vi "Dresden Edit Recipe(in).vi"() -> ()   [LabVIEW 2009] (continued)
          n32 = Scan Value(string=w38, format string="") -> (value=w237:dbl)  [unwired: 1 in, 1 out]
          n33 = Scan Value(string=w40, format string="") -> (value=w249:dbl)  [unwired: 1 in, 1 out]
          n34 = Scan Value(string=w43, format string="") -> (value=w365:dbl)  [unwired: 1 in, 1 out]
          n35 = Scan Value(string=w44, format string="") -> (value=w366:dbl)  [unwired: 1 in, 1 out]
          n36 = Equal?(x="Active", y=w53) -> (x = y?=w134:bool)
          n37 = Scan Value(string=w42, format string="") -> (value=w364:dbl)  [unwired: 1 in, 1 out]
          n38 = Scan Value(string=w35, format string="") -> (value=w231:dbl)  [unwired: 1 in, 1 out]
          n39 = Scan Value(string=w36, format string="") -> (value=w234:dbl)  [unwired: 1 in, 1 out]
          n40 = Scan Value(string=w34, format string="") -> (value=w230:dbl)  [unwired: 1 in, 1 out]
          n41 = Scan Value(string=w56, format string="") -> (value=w387:dbl)  [unwired: 1 in, 1 out]
          n42 = Scan Value(string=w52, format string="") -> (value=w380:dbl)  [unwired: 1 in, 1 out]
          n43 = Scan Value(string=w55, format string="") -> (value=w386:dbl)  [unwired: 1 in, 1 out]
          n44 = case shown="False" w131 {
            frame #0 {
              n45 = local write "Thickness_Monitor_Active"(FALSE ("Thickness_Monitor_Active")) -> ()
            }
            frame #1 {
              n46 = local write "Thickness_Monitor_Active"(TRUE ("Thickness_Monitor_Active")) -> ()
            }
          }
          n47 = Scan Value(string=w51, format string="") -> (value=w379:dbl)  [unwired: 1 in, 1 out]
          n48 = Scan Value(string=w47, format string="") -> (value=w372:dbl)  [unwired: 1 in, 1 out]
          n49 = Scan Value(string=w48, format string="") -> (value=w373:dbl)  [unwired: 1 in, 1 out]
          n50 = case shown="1" w241 {
            frame #0 {
            }
            frame #1 {
              n51 = local write "R_First_stop_selection"(enum32{"Chamber II", "Chamber III"}."Chamber II" ("R_First_stop_selection")) -> ()
            }
            frame #2 {
              n52 = local write "R_First_stop_selection"(enum32{"Chamber II", "Chamber III"}."Chamber III" ("R_First_stop_selection")) -> ()
            }
          }
          n53 = Scan Value(string=w54, format string="") -> (value=w385:dbl)  [unwired: 1 in, 1 out]
          n54 = Scan Value(string=w46, format string="") -> (value=w371:dbl)  [unwired: 1 in, 1 out]
          n55 = case shown="False" w429 {
            frame #0 {
              n56 = local write "R Cmb Step2 Coating Power Active"(FALSE ("R Cmb Step2 Coating Power Active")) -> ()
            }
            frame #1 {
              n57 = local write "R Cmb Step2 Coating Power Active"(TRUE ("R Cmb Step2 Coating Power Active")) -> ()
            }
          }
          n58 = Scan Value(string=w50, format string="") -> (value=w378:dbl)  [unwired: 1 in, 1 out]
          n59 = case shown="False" w421 {
            frame #0 {
              n60 = local write "R Cmb Step3 Coating Power Active"(FALSE ("R Cmb Step3 Coating Power Active")) -> ()
            }
            frame #1 {
              n61 = local write "R Cmb Step3 Coating Power Active"(TRUE ("R Cmb Step3 Coating Power Active")) -> ()
            }
          }
          n62 = Scan Value(string=w60, format string="") -> (value=w394:dbl)  [unwired: 1 in, 1 out]
          n63 = Scan Value(string=w59, format string="") -> (value=w393:dbl)  [unwired: 1 in, 1 out]
          n64 = Equal?(x="Active", y=w45) -> (x = y?=w133:bool)
          n65 = Scan Value(string=w58, format string="") -> (value=w392:dbl)  [unwired: 1 in, 1 out]
          n66 = Equal?(x="Active", y=w49) -> (x = y?=w132:bool)
          n67 = case shown="False" w413 {
            frame #0 {
              n68 = local write "R Cmb Step4 Coating Power Active"(FALSE ("R Cmb Step4 Coating Power Active")) -> ()
            }
            frame #1 {
              n69 = local write "R Cmb Step4 Coating Power Active"(TRUE ("R Cmb Step4 Coating Power Active")) -> ()
            }
          }
          n70 = case shown="False" w405 {
            frame #0 {
              n71 = local write "R Cmb Step5 Coating Power Active"(FALSE ("R Cmb Step5 Coating Power Active")) -> ()
            }
            frame #1 {
              n72 = local write "R Cmb Step5 Coating Power Active"(TRUE ("R Cmb Step5 Coating Power Active")) -> ()
            }
          }
          n73 = case shown="False" w136 {
            frame #0 {
              n74 = local write "R Cmb Step6 Coating Power Active"(FALSE ("R Cmb Step6 Coating Power Active")) -> ()
            }
            frame #1 {
              n75 = local write "R Cmb Step6 Coating Power Active"(TRUE ("R Cmb Step6 Coating Power Active")) -> ()
            }
          }
          n76 = Scan Value(string=w68, format string="") -> (value=w409:dbl)  [unwired: 1 in, 1 out]
          n77 = Scan Value(string=w67, format string="") -> (value=w408:dbl)  [unwired: 1 in, 1 out]
          n78 = Scan Value(string=w64, format string="") -> (value=w401:dbl)  [unwired: 1 in, 1 out]
          n79 = Scan Value(string=w81, format string="") -> (value=w433:dbl)  [unwired: 1 in, 1 out]
          n80 = Scan Value(string=w78, format string="") -> (value=w431:dbl)  [unwired: 1 in, 1 out]
          n81 = Scan Value(string=w63, format string="") -> (value=w400:dbl)  [unwired: 1 in, 1 out]
          n82 = case shown="True" w135 {
            frame #0 {
              n83 = local write "R Cmb Step7 Coating Power Active"(FALSE ("R Cmb Step7 Coating Power Active")) -> ()
            }
            frame #1 {
              n84 = local write "R Cmb Step7 Coating Power Active"(TRUE ("R Cmb Step7 Coating Power Active")) -> ()
            }
          }
          n85 = Scan Value(string=w66, format string="") -> (value=w407:dbl)  [unwired: 1 in, 1 out]
          n86 = Scan Value(string=w80, format string="") -> (value=w432:dbl)  [unwired: 1 in, 1 out]
          n87 = Scan Value(string=w62, format string="") -> (value=w399:dbl)  [unwired: 1 in, 1 out]
          n88 = Scan Value(string=w72, format string="") -> (value=w419:dbl)  [unwired: 1 in, 1 out]
          n89 = Scan Value(string=w71, format string="") -> (value=w416:dbl)  [unwired: 1 in, 1 out]
          n90 = case shown="True" w134 {
            frame #0 {
              n91 = local write "R Cmb Step8 Coating Power Active"(FALSE ("R Cmb Step8 Coating Power Active")) -> ()
            }
            frame #1 {
              n92 = local write "R Cmb Step8 Coating Power Active"(TRUE ("R Cmb Step8 Coating Power Active")) -> ()
            }
          }
          n93 = local write "R Cmb Number of cycle"(w249) -> ()
          n94 = Scan Value(string=w76, format string="") -> (value=w425:dbl)  [unwired: 1 in, 1 out]
          n95 = Scan Value(string=w74, format string="") -> (value=w423:dbl)  [unwired: 1 in, 1 out]
          n96 = Scan Value(string=w70, format string="") -> (value=w415:dbl)  [unwired: 1 in, 1 out]
          n97 = Scan Value(string=w75, format string="") -> (value=w424:dbl)  [unwired: 1 in, 1 out]
          n98 = case shown="True" w133 {
            frame #0 {
              n99 = local write "R Cmb Step10 Coating Power Active"(FALSE ("R Cmb Step10 Coating Power Active")) -> ()
            }
            frame #1 {
              n100 = local write "R Cmb Step10 Coating Power Active"(TRUE ("R Cmb Step10 Coating Power Active")) -> ()
            }
          }
          n101 = local write "R Cmb Ch2 Step10 Coating Power"(w366) -> ()
          n102 = case shown="True" w132 {
            frame #0 {
              n103 = local write "R Cmb Step9 Coating Power Active"(FALSE ("R Cmb Step9 Coating Power Active")) -> ()
            }
            frame #1 {
              n104 = local write "R Cmb Step9 Coating Power Active"(TRUE ("R Cmb Step9 Coating Power Active")) -> ()
            }
          }
          n105 = local write "R Cmb Ch3 Step10 Coating Power"(w365) -> ()
          n106 = local write "R Toooling_factor"(w230) -> ()
          n107 = local write "R Cmb Ch2 Step9 Coating Power"(w373) -> ()
          n108 = local write "R Cmb Ch3 Step9 Coating Power"(w372) -> ()
          n109 = local write "R Cmb Ch3 Step6 Coating Power"(w393) -> ()
          n110 = local write "R Cmb Ch3 Step8 Coating Power"(w379) -> ()
          n111 = local write "R Set Pressure mtorr"(w237) -> ()
          n112 = local write "R Cmb Ch3 Step1 Coating Power"(w432) -> ()
          n113 = local write "R Z_factor"(w231) -> ()
          n114 = local write "R Argon Flow sccm"(w238) -> ()
          n115 = local write "R Cmb Interval length 10"(w364) -> ()
          n116 = local write "R Cmb Ch2 Step7 Coating Power"(w387) -> ()
          n117 = local write "R Cmb Ch3 Step7 Coating Power"(w386) -> ()
          n118 = local write "R Cmb Ch2 Step1 Coating Power"(w433) -> ()
          n119 = local write "R Cmb Interval length 1"(w431) -> ()
          n120 = local write "R Material_density"(w234) -> ()
          n121 = local write "R Cmb Ch2 Step6 Coating Power"(w394) -> ()
          n122 = local write "R Cmb Ch2 Step8 Coating Power"(w380) -> ()
          n123 = local write "R Cmb Ch2 Step5 Coating Power"(w401) -> ()
          n124 = local write "R Cmb Ch3 Step5 Coating Power"(w400) -> ()
          n125 = local write "R Cmb Interval length 9"(w371) -> ()
          n126 = local write "R Cmb Ch2 Step2 Coating Power"(w425) -> ()
          n127 = local write "R Cmb Interval length 8"(w378) -> ()
          n128 = local write "R Cmb Ch3 Step2 Coating Power"(w424) -> ()
          n129 = local write "R Cmb Ch2 Step4 Coating Power"(w409) -> ()
          n130 = local write "R Cmb Ch3 Step3 Coating Power"(w416) -> ()
          n131 = local write "R Cmb Interval length 3"(w415) -> ()
          n132 = local write "R Cmb Interval length 6"(w392) -> ()
          n133 = local write "R Cmb Ch3 Step4 Coating Power"(w408) -> ()
          n134 = local write "R Cmb Interval length 5"(w399) -> ()
          n135 = local write "R Cmb Interval length 7"(w385) -> ()
          n136 = local write "R Cmb Ch2 Step3 Coating Power"(w419) -> ()
          n137 = local write "R Cmb Interval length 2"(w423) -> ()
          n138 = Scan Value(string=w82, format string="") -> (value=w434:dbl)  [unwired: 1 in, 1 out]
          n139 = local write "R Cmb Interval length 4"(w407) -> ()
          n140 = Scan Value(string=w84, format string="") -> (value=w435:dbl)  [unwired: 1 in, 1 out]
          n141 = local write "R Cmb Ch3 Target material"(w83) -> ()
          n142 = local write "R_Cmb_Ch3_Web_speed"(w434) -> ()
          n143 = local write "R Cmb Ch2 Target material"(w23) -> ()
          n144 = local write "R_Cmb_Ch2_Web_speed"(w435) -> ()
          n145 = Equal?(x="Web", y=w519) -> (x = y?=w722:bool)
          n146 = Equal?(x="Other", y=w519) -> (x = y?=w721:bool)
          n147 = Equal?(x="Single", y=w502) -> (x = y?=w689:bool)
          n148 = Equal?(x="Multilayer", y=w502) -> (x = y?=w690:bool)
          n149 = Equal?(x="DC Sputter", y=w511) -> (x = y?=w697:bool)
          n150 = Equal?(x="Microwave Plasma", y=w511) -> (x = y?=w698:bool)
          n151 = Equal?(x="RF Sputter", y=w511) -> (x = y?=w693:bool)
          n152 = Equal?(x="Thickness", y=w512) -> (x = y?=w712:bool)
          n153 = Build Array(FALSE, w722, w721) -> (w726:bool[])
          n154 = Equal?(x="Time", y=w512) -> (x = y?=w713:bool)
          n155 = Equal?(x="Active", y=w88) -> (x = y?=w622:bool)
          n156 = Equal?(x="Active", y=w97) -> (x = y?=w628:bool)
          n157 = Equal?(x="Active", y=w85) -> (x = y?=w439:bool)
          n158 = Equal?(x="Active", y=w257) -> (x = y?=w675:bool)
          n159 = Equal?(x="Active", y=w94) -> (x = y?=w626:bool)
          n160 = Build Array(FALSE, w689, w690) -> (w685:bool[])
          n161 = Boolean Array To Number(Boolean array=w726) -> (number=w725:u32)
          n162 = Equal?(x="Active", y=w103) -> (x = y?=w632:bool)
          n163 = Equal?(x="Active", y=w100) -> (x = y?=w630:bool)
          n164 = Build Array(FALSE, w698, w697, w693) -> (w702:bool[])
          n165 = Equal?(x="Active", y=w117) -> (x = y?=w656:bool)
          n166 = Equal?(x="Active", y=w115) -> (x = y?=w653:bool)
          n167 = Equal?(x="Chamber III", y=w272) -> (x = y?=w602:bool)
          n168 = Equal?(x="Chamber II", y=w272) -> (x = y?=w603:bool)
          n169 = Equal?(x="Active", y=w112) -> (x = y?=w644:bool)
          n170 = Equal?(x="Active", y=w124) -> (x = y?=w660:bool)
          n171 = Equal?(x="Active", y=w127) -> (x = y?=w672:bool)
          n172 = Equal?(x="Active", y=w121) -> (x = y?=w657:bool)
          n173 = Equal?(x="Active", y=w91) -> (x = y?=w623:bool)
          n174 = Equal?(x="Active", y=w130) -> (x = y?=w662:bool)
          n175 = Equal?(x="Active", y=w106) -> (x = y?=w636:bool)
          n176 = Mantissa & Exponent(0:w725) -> (2:w720:dbl)  [unwired: 1 out]
          n177 = Scan Value(string=w99, format string="") -> (value=w31:dbl)  [unwired: 1 in, 1 out]
          n178 = case shown="True" w628 {
            frame #0 {
              n179 = local write "R Single RF Step7 Coating Power Active"(FALSE ("R Single RF Step7 Coating Power Active")) -> ()
            }
            frame #1 {
              n180 = local write "R Single RF Step7 Coating Power Active"(TRUE ("R Single RF Step7 Coating Power Active")) -> ()
            }
          }
          n181 = Scan Value(string=w98, format string="") -> (value=w30:dbl)  [unwired: 1 in, 1 out]
          n182 = Equal?(x="Active", y=w109) -> (x = y?=w640:bool)
          n183 = Scan Value(string=w102, format string="") -> (value=w455:dbl)  [unwired: 1 in, 1 out]
          n184 = Scan Value(string=w101, format string="") -> (value=w454:dbl)  [unwired: 1 in, 1 out]
          n185 = Scan Value(string=w89, format string="") -> (value=w445:dbl)  [unwired: 1 in, 1 out]
          n186 = Scan Value(string=w90, format string="") -> (value=w446:dbl)  [unwired: 1 in, 1 out]
          n187 = Boolean Array To Number(Boolean array=w685) -> (number=w686:u32)
          n188 = Build Array(FALSE, w712, w713) -> (w708:bool[])
          n189 = Scan Value(string=w96, format string="") -> (value=w453:dbl)  [unwired: 1 in, 1 out]
          n190 = Equal?(x="Active", y=w253) -> (x = y?=w666:bool)
          n191 = case shown="True" w630 {
            frame #0 {
              n192 = local write "R Single RF Step6 Coating Power Active"(FALSE ("R Single RF Step6 Coating Power Active")) -> ()
            }
            frame #1 {
              n193 = local write "R Single RF Step6 Coating Power Active"(TRUE ("R Single RF Step6 Coating Power Active")) -> ()
            }
          }
          n194 = Scan Value(string=w93, format string="") -> (value=w449:dbl)  [unwired: 1 in, 1 out]
          n195 = Scan Value(string=w95, format string="") -> (value=w452:dbl)  [unwired: 1 in, 1 out]
          n196 = case shown="True" w626 {
            frame #0 {
              n197 = local write "R Single RF Step8 Coating Power Active"(FALSE ("R Single RF Step8 Coating Power Active")) -> ()
            }
            frame #1 {
              n198 = local write "R Single RF Step8 Coating Power Active"(TRUE ("R Single RF Step8 Coating Power Active")) -> ()
            }
          }
          n199 = Scan Value(string=w92, format string="") -> (value=w448:dbl)  [unwired: 1 in, 1 out]
          n200 = Boolean Array To Number(Boolean array=w702) -> (number=w701:u32)
          n201 = case shown="True" w632 {
            frame #0 {
              n202 = local write "R Single RF Step5 Coating Power Active"(FALSE ("R Single RF Step5 Coating Power Active")) -> ()
            }
            frame #1 {
              n203 = local write "R Single RF Step5 Coating Power Active"(TRUE ("R Single RF Step5 Coating Power Active")) -> ()
            }
          }
          n204 = case shown="False" w622 {
            frame #0 {
              n205 = local write "R Single RF Step10 Coating Power Active"(FALSE ("R Single RF Step10 Coating Power Active")) -> ()
            }
            frame #1 {
              n206 = local write "R Single RF Step10 Coating Power Active"(TRUE ("R Single RF Step10 Coating Power Active")) -> ()
            }
          }
          n207 = case shown="False" w623 {
            frame #0 {
              n208 = local write "R Single RF Step9 Coating Power Active"(FALSE ("R Single RF Step9 Coating Power Active")) -> ()
            }
            frame #1 {
              n209 = local write "R Single RF Step9 Coating Power Active"(TRUE ("R Single RF Step9 Coating Power Active")) -> ()
            }
          }
          n210 = Scan Value(string=w86, format string="") -> (value=w441:dbl)  [unwired: 1 in, 1 out]
          n211 = Scan Value(string=w122, format string="") -> (value=w470:dbl)  [unwired: 1 in, 1 out]
          n212 = Scan Value(string=w87, format string="") -> (value=w442:dbl)  [unwired: 1 in, 1 out]
          n213 = Scan Value(string=w123, format string="") -> (value=w471:dbl)  [unwired: 1 in, 1 out]
          n214 = case shown="True" w656 {
            frame #0 {
              n215 = local write "R Single RF Ramp up"(FALSE ("R Single RF Ramp up")) -> ()
            }
            frame #1 {
              n216 = local write "R Single RF Ramp up"(TRUE ("R Single RF Ramp up")) -> ()
            }
          }
          n217 = Scan Value(string=w116, format string="") -> (value=w465:dbl)  [unwired: 1 in, 1 out]
          n218 = case shown="False" w653 {
            frame #0 {
              n219 = local write "R Single RF Step1 Coating Power Active"(FALSE ("R Single RF Step1 Coating Power Active")) -> ()
            }
            frame #1 {
              n220 = local write "R Single RF Step1 Coating Power Active"(TRUE ("R Single RF Step1 Coating Power Active")) -> ()
            }
          }
          n221 = Scan Value(string=w125, format string="") -> (value=w472:dbl)  [unwired: 1 in, 1 out]
          n222 = Scan Value(string=w128, format string="") -> (value=w474:dbl)  [unwired: 1 in, 1 out]
          n223 = Scan Value(string=w126, format string="") -> (value=w473:dbl)  [unwired: 1 in, 1 out]
          n224 = Scan Value(string=w129, format string="") -> (value=w475:dbl)  [unwired: 1 in, 1 out]
          n225 = Scan Value(string=w107, format string="") -> (value=w458:dbl)  [unwired: 1 in, 1 out]
          n226 = Scan Value(string=w119, format string="") -> (value=w467:dbl)  [unwired: 1 in, 1 out]
          n227 = case shown="True" w636 {
            frame #0 {
              n228 = local write "R Single RF Step4 Coating Power Active"(FALSE ("R Single RF Step4 Coating Power Active")) -> ()
            }
            frame #1 {
              n229 = local write "R Single RF Step4 Coating Power Active"(TRUE ("R Single RF Step4 Coating Power Active")) -> ()
            }
          }
          n230 = Scan Value(string=w120, format string="") -> (value=w468:dbl)  [unwired: 1 in, 1 out]
          n231 = case shown="True" w644 {
            frame #0 {
              n232 = local write "R Single RF Step2 Coating Power Active"(FALSE ("R Single RF Step2 Coating Power Active")) -> ()
            }
            frame #1 {
              n233 = local write "R Single RF Step2 Coating Power Active"(TRUE ("R Single RF Step2 Coating Power Active")) -> ()
            }
          }
          n234 = Scan Value(string=w108, format string="") -> (value=w459:dbl)  [unwired: 1 in, 1 out]
          n235 = local write "R Single DC Target material"(w270) -> ()
          n236 = case shown="True" w672 {
            frame #0 {
              n237 = local write "R Single DC Step8 Coating Power Active"(FALSE ("R Single DC Step8 Coating Power Active")) -> ()
            }
            frame #1 {
              n238 = local write "R Single DC Step8 Coating Power Active"(TRUE ("R Single DC Step8 Coating Power Active")) -> ()
            }
          }
          n239 = Scan Value(string=w114, format string="") -> (value=w464:dbl)  [unwired: 1 in, 1 out]
          n240 = Scan Value(string=w113, format string="") -> (value=w463:dbl)  [unwired: 1 in, 1 out]
          n241 = Scan Value(string=w110, format string="") -> (value=w460:dbl)  [unwired: 1 in, 1 out]
          n242 = Equal?(x="Active", y=w260) -> (x = y?=w676:bool)
          n243 = case shown="True" w657 {
            frame #0 {
              n244 = local write "R Single DC Step10 Coating Power Active"(FALSE ("R Single DC Step10 Coating Power Active")) -> ()
            }
            frame #1 {
              n245 = local write "R Single DC Step10 Coating Power Active"(TRUE ("R Single DC Step10 Coating Power Active")) -> ()
            }
          }
          n246 = case shown="False" w439 {
            frame #0 {
              n247 = local write "R Single RF Ramp down"(FALSE ("R Single RF Ramp down")) -> ()
            }
            frame #1 {
              n248 = local write "R Single RF Ramp down"(TRUE ("R Single RF Ramp down")) -> ()
            }
          }
          n249 = Mantissa & Exponent(0:w686) -> (2:w691:dbl)  [unwired: 1 out]
          n250 = Scan Value(string=w111, format string="") -> (value=w461:dbl)  [unwired: 1 in, 1 out]
          n251 = case shown="True" w640 {
            frame #0 {
              n252 = local write "R Single RF Step3 Coating Power Active"(FALSE ("R Single RF Step3 Coating Power Active")) -> ()
            }
            frame #1 {
              n253 = local write "R Single RF Step3 Coating Power Active"(TRUE ("R Single RF Step3 Coating Power Active")) -> ()
            }
          }
          n254 = case shown="False" w660 {
            frame #0 {
              n255 = local write "R Single DC Step9 Coating Power Active"(FALSE ("R Single DC Step9 Coating Power Active")) -> ()
            }
            frame #1 {
              n256 = local write "R Single DC Step9 Coating Power Active"(TRUE ("R Single DC Step9 Coating Power Active")) -> ()
            }
          }
          n257 = case shown="False" w662 {
            frame #0 {
              n258 = local write "R Single DC Step7 Coating Power Active"(FALSE ("R Single DC Step7 Coating Power Active")) -> ()
            }
            frame #1 {
              n259 = local write "R Single DC Step7 Coating Power Active"(TRUE ("R Single DC Step7 Coating Power Active")) -> ()
            }
          }
          n260 = local write "R Single RF Target material"(w118) -> ()
          n261 = Scan Value(string=w105, format string="") -> (value=w457:dbl)  [unwired: 1 in, 1 out]
          n262 = Scan Value(string=w104, format string="") -> (value=w456:dbl)  [unwired: 1 in, 1 out]
          n263 = Mantissa & Exponent(0:w701) -> (2:w695:dbl)  [unwired: 1 out]
          n264 = Boolean Array To Number(Boolean array=w708) -> (number=w709:u32)
          n265 = Scan Value(string=w252, format string="") -> (value=w477:dbl)  [unwired: 1 in, 1 out]
          n266 = Scan Value(string=w29, format string="") -> (value=w438:dbl)  [unwired: 1 in, 1 out]
          n267 = Scan Value(string=w268, format string="") -> (value=w489:dbl)  [unwired: 1 in, 1 out]
          n268 = Scan Value(string=w255, format string="") -> (value=w479:dbl)  [unwired: 1 in, 1 out]
          n269 = Scan Value(string=w251, format string="") -> (value=w476:dbl)  [unwired: 1 in, 1 out]
          n270 = Scan Value(string=w256, format string="") -> (value=w480:dbl)  [unwired: 1 in, 1 out]
          n271 = Scan Value(string=w22, format string="") -> (value=w490:dbl)  [unwired: 1 in, 1 out]
          n272 = local write "R Single RF Interval length6"(w30) -> ()
          n273 = case shown="False" w675 {
            frame #0 {
              n274 = local write "R Single DC Step5 Coating Power Active"(FALSE ("R Single DC Step5 Coating Power Active")) -> ()
            }
            frame #1 {
              n275 = local write "R Single DC Step5 Coating Power Active"(TRUE ("R Single DC Step5 Coating Power Active")) -> ()
            }
          }
          n276 = case shown="True" w666 {
            frame #0 {
              n277 = local write "R Single DC Step6 Coating Power Active"(FALSE ("R Single DC Step6 Coating Power Active")) -> ()
            }
            frame #1 {
              n278 = local write "R Single DC Step6 Coating Power Active"(TRUE ("R Single DC Step6 Coating Power Active")) -> ()
            }
          }
          n279 = Scan Value(string=w273, format string="") -> (value=w492:dbl)  [unwired: 1 in, 1 out]
          n280 = local write "R Single RF Step6 Coating Power"(w31) -> ()
          n281 = Scan Value(string=w258, format string="") -> (value=w481:dbl)  [unwired: 1 in, 1 out]
          n282 = Scan Value(string=w259, format string="") -> (value=w482:dbl)  [unwired: 1 in, 1 out]
          n283 = Scan Value(string=w266, format string="") -> (value=w488:dbl)  [unwired: 1 in, 1 out]
          n284 = Scan Value(string=w275, format string="") -> (value=w491:dbl)  [unwired: 1 in, 1 out]
          n285 = Scan Value(string=w274, format string="") -> (value=w493:dbl)  [unwired: 1 in, 1 out]
          n286 = local write "R Single RF Interval length9"(w445) -> ()
          n287 = Scan Value(string=w265, format string="") -> (value=w487:dbl)  [unwired: 1 in, 1 out]
          n288 = local write "R Single RF Step9 Coating Power"(w446) -> ()
          n289 = local write "R Single RF Interval length7"(w452) -> ()
          n290 = local write "R Single RF Step8 Coating Power"(w449) -> ()
          n291 = Scan Value(string=w262, format string="") -> (value=w485:dbl)  [unwired: 1 in, 1 out]
          n292 = local write "R Single RF Interval length8"(w448) -> ()
          n293 = local write "R Single RF Step7 Coating Power"(w453) -> ()
          n294 = Scan Value(string=w261, format string="") -> (value=w484:dbl)  [unwired: 1 in, 1 out]
          n295 = local write "R Single DC Step9 Coating Power"(w471) -> ()
          n296 = local write "R Single RF Ramp up Time"(w465) -> ()
          n297 = local write "R Single RF  Step1 Coating Power"(w464) -> ()
          n298 = local write "R Single RF Step10 Coating Power"(w442) -> ()
          n299 = Mantissa & Exponent(0:w709) -> (2:w706:dbl)  [unwired: 1 out]
          n300 = local write "R Single RF Interval length5"(w454) -> ()
          n301 = local write "R Single RF Interval length10"(w441) -> ()
          n302 = local write "R Single RF Interval length"(w463) -> ()
          n303 = Equal?(x="Active", y=w263) -> (x = y?=w264:bool)
          n304 = local write "R Single RF Step5 Coating Power"(w455) -> ()
          n305 = Build Array(FALSE, w603, w602) -> (w607:bool[])
          n306 = local write "R Single DC Interval length9"(w470) -> ()
          n307 = local write "R Single DC Step10 Coating Power"(w468) -> ()
          n308 = local write "R Single DC Interval length10"(w467) -> ()
          n309 = local write "R Single DC Interval length5"(w479) -> ()
          n310 = case shown="2" w695 {
            frame #0 {
            }
            frame #1 {
              n311 = property on="Single_DC_power_power_tab" class="TabCtl (strict)"("Visible"=FALSE) -> ()  [unwired: 2 in, 2 out]
              n312 = local write "R_Simple_Coating Type Selection"(T2."Microwave Plasma" ("R_Simple_Coating Type Selection")) -> ()
              n313 = property on="Single_RF_power_power_tab" class="TabCtl (strict)"("Visible"=FALSE) -> ()  [unwired: 2 in, 2 out]
            }
            frame #2 {
              n314 = property on="Single_DC_power_power_tab" class="TabCtl (strict)"("Visible"=TRUE) -> ()  [unwired: 2 in, 2 out]
              n315 = local write "R_Simple_Coating Type Selection"(T2."DC Sputter" ("R_Simple_Coating Type Selection")) -> ()
              n316 = local write "Power_singledc_list_open"(TRUE ("Power_singledc_list_open")) -> ()
            }
            frame #3 {
              n317 = property on="Single_RF_power_power_tab" class="TabCtl (strict)"("Visible"=TRUE) -> ()  [unwired: 2 in, 2 out]
              n318 = local write "R_Simple_Coating Type Selection"(T2."RF Sputter" ("R_Simple_Coating Type Selection")) -> ()
              n319 = local write "Power_single_rf_list_open"(TRUE ("Power_single_rf_list_open")) -> ()
            }
          }
          n320 = local write "R Single DC Step7 Coating Power"(w475) -> ()
          n321 = local write "R Single RF Ramp down Time"(w438) -> ()
          n322 = local write "R Single RF Step2 Coating Power"(w461) -> ()
          n323 = local write "R Single DC Step1 Coating Power"(w489) -> ()
          n324 = local write "R Single RF Interval length2"(w460) -> ()
          n325 = local write "R Single DC Step5 Coating Power"(w480) -> ()
          n326 = case shown="2" w720 {
            frame #0 {
            }
            frame #1 {
              n327 = local write "R_Web_selection"(enum32{"Web", "Other"}."Web" ("R_Web_selection")) -> ()
            }
            frame #2 {
              n328 = local write "R_Web_selection"(enum32{"Web", "Other"}."Other" ("R_Web_selection")) -> ()
            }
          }
          n329 = local write "R Single DC Interval length7"(w474) -> ()
          n330 = case shown="False" w676 {
            frame #0 {
              n331 = local write "R Single DC Step4 Coating Power Active"(FALSE ("R Single DC Step4 Coating Power Active")) -> ()
            }
            frame #1 {
              n332 = local write "R Single DC Step4 Coating Power Active"(TRUE ("R Single DC Step4 Coating Power Active")) -> ()
            }
          }
          n333 = local write "R Single DC Step8 Coating Power"(w473) -> ()
          n334 = local write "R Single RF Step3 Coating Power"(w459) -> ()
          n335 = local write "R Single RF Interval length3"(w458) -> ()
          n336 = local write "R Single RF Step4 Coating Power"(w457) -> ()
          n337 = local write "R Single RF Interval length4"(w456) -> ()
          n338 = local write "R Single DC Interval length8"(w472) -> ()
          n339 = local write "R Single DC Step6 Coating Power"(w477) -> ()
          n340 = local write "R Single DC Interval length1"(w490) -> ()
          n341 = case shown="1" w706 {
            frame #0 {
            }
            frame #1 {
              n342 = local write "R_Thickness Selection"(enum32{"Thickness", "Time"}."Thickness" ("R_Thickness Selection")) -> ()
            }
            frame #2 {
              n343 = local write "R_Thickness Selection"(enum32{"Thickness", "Time"}."Time" ("R_Thickness Selection")) -> ()
            }
          }
          n344 = local write "R Single DC Step4 Coating Power"(w482) -> ()
          n345 = local write "R Single DC Interval length2"(w487) -> ()
          n346 = local write "R Single DC Interval length6"(w476) -> ()
          n347 = local write "R_Single Microwave Time"(w493) -> ()
          n348 = local write "R Single DC Step3 Coating Power"(w485) -> ()
          n349 = local write "R_Single Microwave Power"(w491) -> ()
          n350 = Boolean Array To Number(Boolean array=w607) -> (number=w608:u32)
          n351 = local write "R Single DC Interval length4"(w481) -> ()
          n352 = local write "R Single Pass Number"(w492) -> ()
          n353 = local write "R Single DC Step2 Coating Power"(w488) -> ()
          n354 = local write "R Single DC Interval length3"(w484) -> ()
          n355 = case shown="True" w264 {
            frame #0 {
              n356 = local write "R Single DC Step3 Coating Power Active"(FALSE ("R Single DC Step2 Coating Power Active")) -> ()
            }
            frame #1 {
              n357 = local write "R Single DC Step3 Coating Power Active"(TRUE ("R Single DC Step2 Coating Power Active")) -> ()
            }
          }
          n358 = Scan Value(string=w517, format string="") -> (value=w500:dbl)  [unwired: 1 in, 1 out]
          n359 = Scan Value(string=w516, format string="") -> (value=w499:dbl)  [unwired: 1 in, 1 out]
          n360 = Scan Value(string=w518, format string="") -> (value=w501:dbl)  [unwired: 1 in, 1 out]
          n361 = Scan Value(string=w515, format string="") -> (value=w498:dbl)  [unwired: 1 in, 1 out]
          n362 = Scan Value(string=w513, format string="") -> (value=w496:dbl)  [unwired: 1 in, 1 out]
          n363 = Scan Value(string=w24, format string="") -> (value=w495:dbl)  [unwired: 1 in, 1 out]
          n364 = Scan Value(string=w276, format string="") -> (value=w494:dbl)  [unwired: 1 in, 1 out]
          n365 = Scan Value(string=w514, format string="") -> (value=w497:dbl)  [unwired: 1 in, 1 out]
          n366 = Equal?(x="Active", y=w21) -> (x = y?=w271:bool)
          n367 = case shown="2" w691 {
            frame #0 {
            }
            frame #1 {
              n368 = local write "R_Recipe_type_selection"(enum32{"Single Recipe", "Combination Sputter"}."Single Recipe" ("R_Recipe_type_selection")) -> ()
              n369 = property on="Multilayer_power_tab" class="TabCtl (strict)"("Visible"=FALSE) -> ()  [unwired: 2 in, 2 out]
            }
            frame #2 {
              n370 = local write "Power_list_open_multi"(TRUE ("Power_list_open_multi")) -> ()
              n371 = property on="Multilayer_power_tab" class="TabCtl (strict)"("Visible"=TRUE) -> ()  [unwired: 2 in, 2 out]
